vi "RewindMusic.vi"(0 "reference in":refnum<class "MediaPlayer.lvclass">, 11 "Error In":errorcluster) -> (4 "reference out":refnum<class "MediaPlayer.lvclass">, 15 "Error Out":errorcluster)   [LabVIEW 2024, in "MediaPlayer.lvclass"]
doc: "Goes back to song one before the current one"
uses:
  MediaPlayer.lvclass
panel:
  # "Connector Pane"
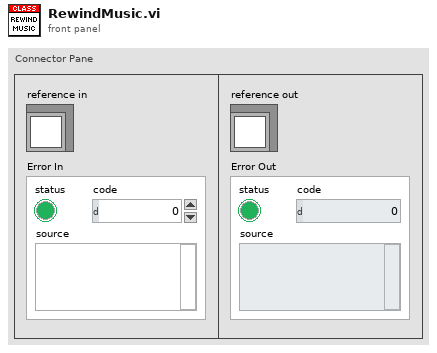
[diagram p1: front panel]
types:
  T1 = typedef "MediaPlayer.lvclass/ObjectAttributes.ctl" = cluster{"MediaPlayerData":T2, "Current Info":T4}
  T2 = typedef "MediaPlayer.lvclass/MediaPlayer Data.ctl" = cluster{"Music List":path[], "Current Music Index":i64, "Song Handler":T3, "Device ID":u32}
  T3 = typedef "Sound Output Task ID.ctl" = u32
  T4 = typedef "MediaPlayer.lvclass/Current Info.ctl" = cluster{"Duration":dbl, "Name":string, "Is playing?":bool, "Current Music Index":i64}
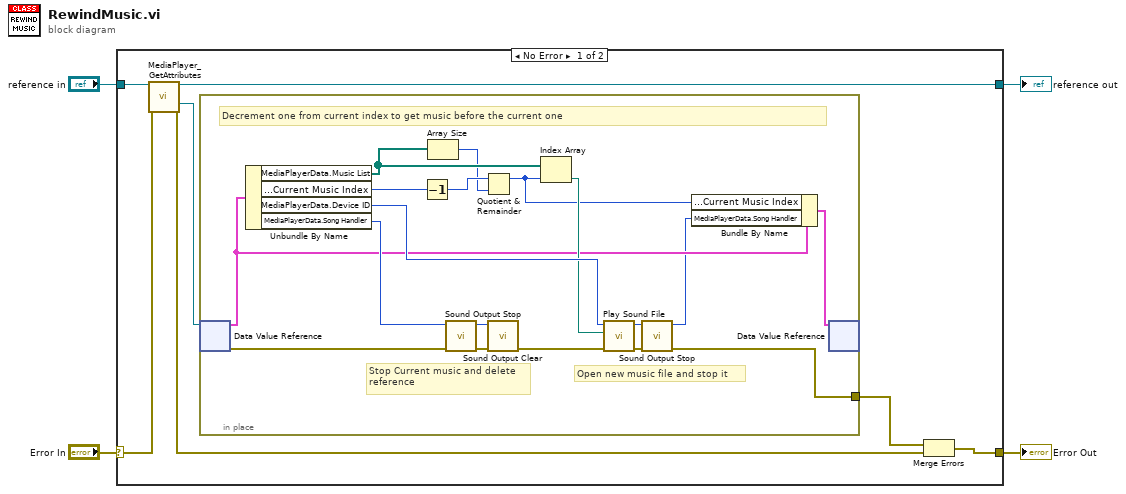
[diagram p0: block diagram]
diagram:
  n1 = case shown="No Error" "Error In" {
    selector: "Error In" -> [w11 w31]
    tunnel: [w6 w31] -> w3
    tunnel: [w8 w30] -> w1
    tunnel: "reference in" -> [w9 w30]
    frame No Error {
      n2 = call "MediaPlayer_GetAttributes.vi"("reference in"=w9, "Error In"=w11) -> ("reference out"=w8:refnum<class "MediaPlayer.lvclass">, "DataRef"=w7:refnum<data-value>, "Error Out"=w10:errorcluster)  [unwired: 10 in, 1 out]
      n3 = in-place {
        in-place-border: [w15] -> w5
        # "Decrement one from current index to get music before the current one"
        # "Open new music file and stop it"
        # "Stop Current music and delete\nreference"
        n4 = in-place-dvr #1(w7) -> (w18:T1, w26:errorcluster)
        n5 = Unbundle By Name(w18) -> ("MediaPlayerData.Music List"=w28:path[], "MediaPlayerData.Current Music Index"=w29:i64, "MediaPlayerData.Device ID"=w22:u32, "MediaPlayerData.Song Handler"=w27:T3)
        n6 = Decrement(x=w29) -> (x-1=w14:i64)
        n7 = Array Size(array=w28) -> (size(s)=w13:i32)
        n8 = call <vilib>:"Sound Output Stop.vi"("error in (no error)"=w26, "task ID"=w27) -> ("error out"=w25:errorcluster, "task ID out"=w24:T3)  [unwired: 8 in]
        n9 = Quotient & Remainder(x=w14, y=w13) -> (x-y*floor(x/y)=w12:i64)  [unwired: 1 out]
        n10 = call <vilib>:"Sound Output Clear.vi"("error in (no error)"=w25, "task ID"=w24) -> ("error out"=w23:errorcluster)  [unwired: 9 in]
        n11 = Index Array(array=w28, index=w12) -> (element=w21:path)
        n12 = call <vilib>:"Play Sound File.vi"("error in (no error)"=w23, "path"=w21, "device ID"=w22) -> ("error out"=w20:errorcluster, "task ID"=w19:T3)  [unwired: 7 in]
        n13 = call <vilib>:"Sound Output Stop.vi"("error in (no error)"=w20, "task ID"=w19) -> ("error out"=w15:errorcluster, "task ID out"=w17:T3)  [unwired: 8 in]
        n14 = Bundle By Name(cluster=w18, "MediaPlayerData.Current Music Index"=w12, "MediaPlayerData.Song Handler"=w17) -> (w16:T1)
        n15 = in-place-dvr #1(w16) -> ()  [unwired: 2 out]
      }
      n16 = Merge Errors(w5, w10) -> (w6:errorcluster)
    }
    frame Error {
    }
  }
  "Error Out" <- w3
  "reference out" <- w1
